vi "LensMotorsS3_move.vi"(8 "error in (no error)":errorcluster, 10 "delta":sgl, 11 "channel":refnum<k24>) -> (0 "error out":errorcluster)   [LabVIEW 2021]
uses:
  F:/2PhotonVision/psychometric_function_v2/lib/Grpc.Core.dll
  lib/Grpc.Core.dll
  F:/2PhotonVision/psychometric_function_v2/lib/FossilProtosSharp.dll
  lib/FossilProtosSharp.dll
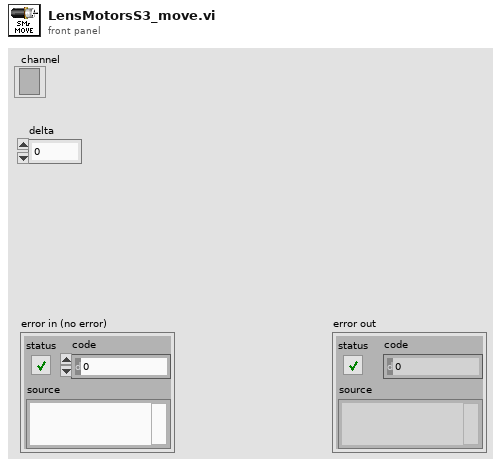
[diagram p1: front panel]
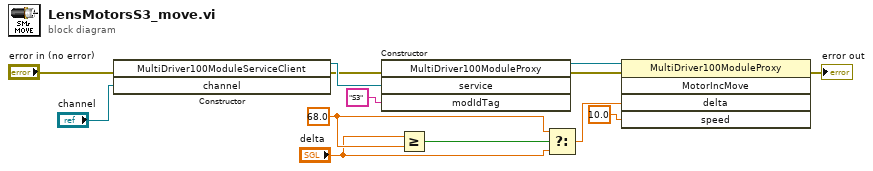
[diagram p0: block diagram]
diagram:
  w7 = sgl 68.0 ("y")
  n1 = constructor class="MultiDriver100ModuleServiceClie"(error in="error in (no error)", "channel"="channel") -> (reference out=w11:refnum<k24>, error out=w10:errorcluster)  [unwired: 2 in, 2 out]
  n2 = constructor class="MultiDriver100ModuleProxy"(error in=w10, "service"=w11, "modIdTag"="S3") -> (reference out=w5:refnum<k24>, error out=w6:errorcluster)  [unwired: 2 in, 3 out]
  n3 = Greater Or Equal?(x="delta", y=w7) -> (x >= y?=w9:bool)
  n4 = Select(t=w7, s=w9, f="delta") -> (s? t:f=w3:sgl)
  n5 = invoke class="MultiDriver100ModuleProxy" method="MotorIncMove"(reference=w5, error in=w6, "delta"=w3, "speed"=sgl 10.0) -> (error out=→"error out":errorcluster)  [unwired: 1 in, 4 out]
